vi "unused_getType.vi"(8 "error in (no error)":errorcluster, 11 "BlockDiagram In":refnum<class "BlockDiagram.lvclass">) -> (0 "error out":errorcluster, 2 "type":refnum<vi>, 3 "BlockDiagram Out":refnum<class "BlockDiagram.lvclass">)   [LabVIEW 2023]
uses:
  BlockDiagram.lvclass/BlockDiagram.ctl
  BlockDiagram.lvclass
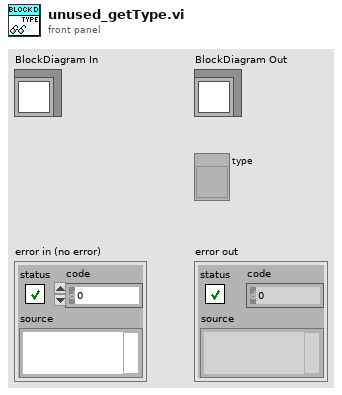
[diagram p1: front panel]
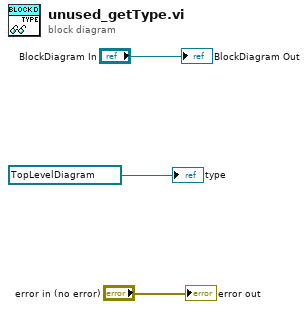
[diagram p0: block diagram]
diagram:
  "error out" <- "error in (no error)"
  "BlockDiagram Out" <- "BlockDiagram In"
  "type" <- refnum<vi> refnum ("Reference to Diagram")
